vi "Tag Name.vi"() -> (3 "String":string="DataGridQControlConfig")   [LabVIEW 2018, in "DataGrid Config.lvclass"]
uses:
  DataGrid Config.lvclass
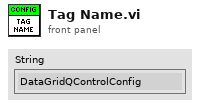
[diagram p1: front panel]
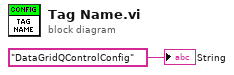
[diagram p0: block diagram]
diagram:
  "String" <- "DataGridQControlConfig"
